vi "Agilent VNA Determine Next Trace.vi"(7 "Reset?":bool, 10 "Channel":i8) -> (2 "Next Trace":i8)   [LabVIEW 2011]
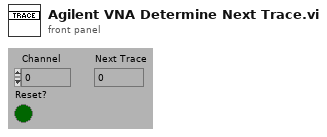
[diagram p1: front panel]
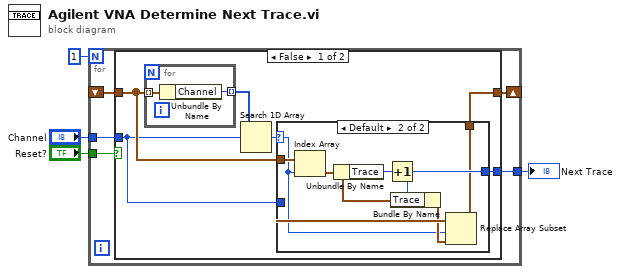
[diagram p0: block diagram]
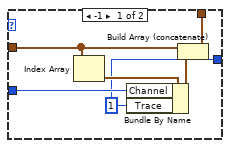
[diagram p2: hidden frame]
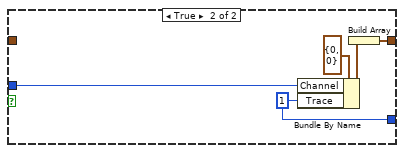
[diagram p3: hidden frame]
diagram:
  n1 = for {
    N: 1 -> [_]
    shift-right: [w7] -> _
    shift-left: _ -> [w8]
    tunnel: "Channel" -> [w6]
    tunnel: [w9] -> w3
    tunnel: "Reset?" -> [w5]
    n2 = case shown="False" w5 {
      tunnel: [w14 w34] -> w9
      tunnel: w8 -> [w13 _]
      tunnel: [w12 w32] -> w7
      tunnel: w6 -> [w10 w31]
      frame False {
        n3 = for {
          tunnel: w13 -> [w30] mode=indexing
          tunnel: [w29] -> w15 mode=indexing
          n4 = Unbundle By Name(w30) -> ("Channel"=w29:i8)
        }
        n5 = Search 1D Array(1D array=w15, element=w10) -> (index of element=w11:i32)  [unwired: 1 out]
        n6 = case shown="Default" w11 {
          selector: w11 -> [_ w22]
          tunnel: [w16 w26] -> w14
          tunnel: w13 -> [w20 w25]
          tunnel: [w21 w23] -> w12
          tunnel: w10 -> [w17 _]
          frame -1 {
            w16 = i8 1 ("Trace")
            n7 = Index Array(array=w20) -> (element=w19:cluster{"Channel":i8, "Trace":i8})  [unwired: 1 in]
            n8 = Bundle By Name(cluster=w19, "Channel"=w17, "Trace"=w16) -> (w18:cluster{"Channel":i8, "Trace":i8})
            n9 = Build Array (concatenate)(w20, w18) -> (w21:cluster{"Channel":i8, "Trace":i8}[])
          }
          frame Default {
            n10 = Index Array(array=w25, index=w22) -> (element=w27:cluster{"Channel":i8, "Trace":i8})
            n11 = Unbundle By Name(w27) -> ("Trace"=w28:i8)
            n12 = Increment(x=w28) -> (x+1=w26:i8)
            n13 = Bundle By Name(cluster=w27, "Trace"=w26) -> (w24:cluster{"Channel":i8, "Trace":i8})
            n14 = Replace Array Subset(array=w25, new element=w24, index=w22) -> (w23:cluster{"Channel":i8, "Trace":i8}[])
          }
        }
      }
      frame True {
        w34 = i8 1 ("Trace")
        n15 = Bundle By Name(cluster=cluster{"Channel":i8, "Trace":i8} {"Channel"=0, "Trace"=0}, "Channel"=w31, "Trace"=w34) -> (w35:cluster{"Channel":i8, "Trace":i8})
        n16 = Build Array(w35) -> (w32:cluster{"Channel":i8, "Trace":i8}[])
      }
    }
  }
  "Next Trace" <- w3
